vi "Rx Async.vi"(8 "error in (no error)":errorcluster, 10 "Dispatcher Interface in":refnum<class "Dispatcher Interface.lvclass">, 11 "Plugin in":refnum<class "Plugin.lvclass">) -> (0 "error out":errorcluster, 2 "Dispatcher Interface out":refnum<class "Dispatcher Interface.lvclass">, 3 "Plugin out":refnum<class "Plugin.lvclass">)   [LabVIEW 2017, in "DSF Core.lvlib" / "Plugin.lvclass"]
uses:
  Plugin.lvclass
  Interface/Dispatcher/Dispatcher Interface.lvclass
  Plugin.lvclass/Plugin.ctl
  Interface/Dispatcher/Command.ctl
  Transfer Group/Transfer Group.lvclass
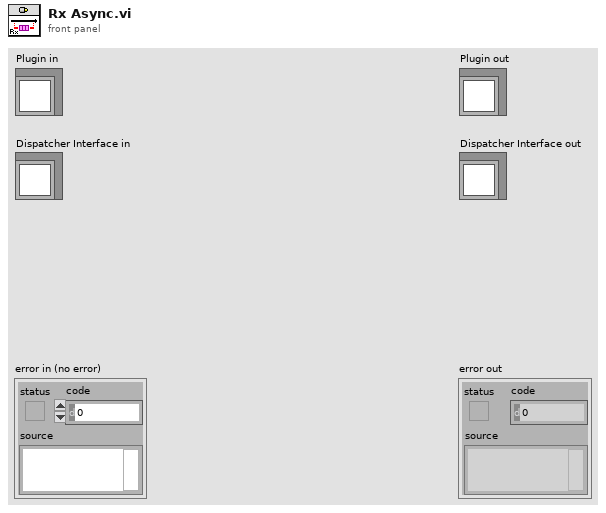
[diagram p1: front panel]
types:
  T1 = typedef "DSF Core.lvlib/Dispatcher Interface.lvclass/Command.ctl" = enum8{"Idle", "Start", "Rx", "Tx", "Set Inline Buffer", "Shutdown", "Error"}
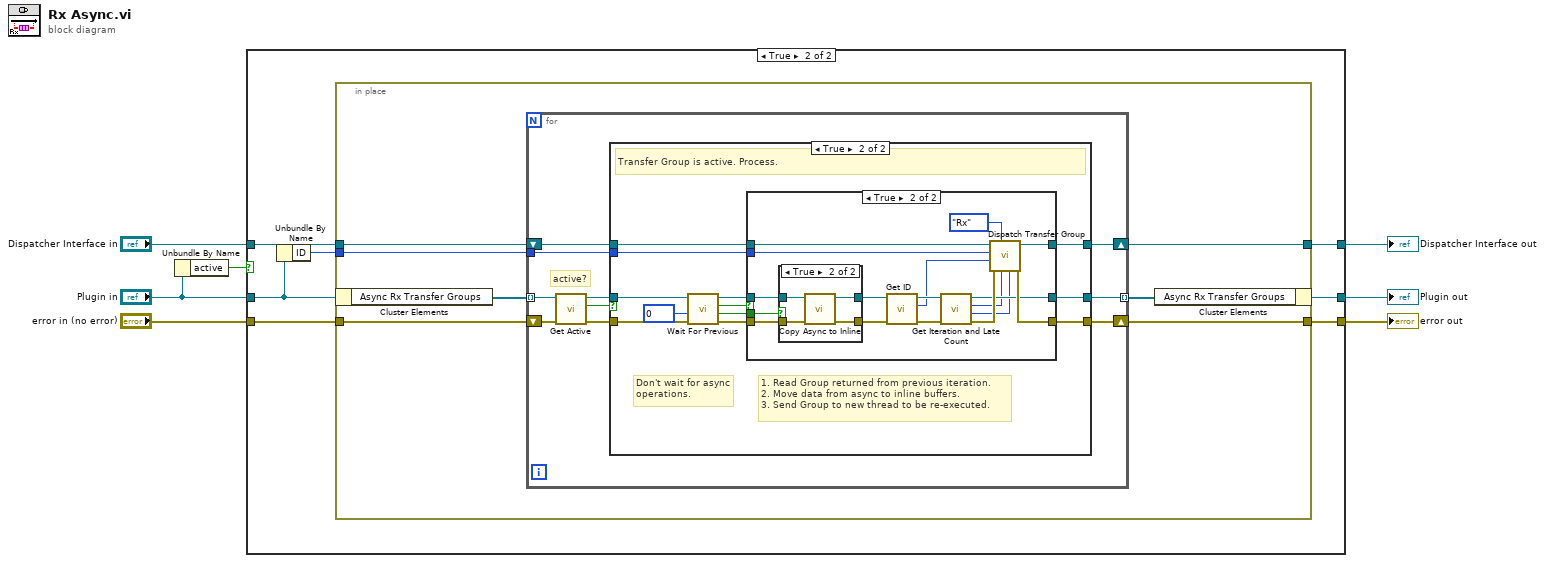
[diagram p0: block diagram]
diagram:
  n1 = Unbundle By Name("Plugin in") -> ("active"=w1:bool)
  n2 = case shown="True" w1 {
    tunnel: "error in (no error)" -> [w8 w17]
    tunnel: [w8 w16] -> w6
    tunnel: [w10 w15] -> w5
    tunnel: "Dispatcher Interface in" -> [w9 w14]
    tunnel: [w9 w13] -> w3
    tunnel: "Plugin in" -> [w10 w12]
    frame False {
    }
    frame True {
      n3 = Unbundle By Name(w12) -> ("ID"=w11:i32)
      n4 = in-place {
        in-place-border: w17 -> [w24]
        in-place-border: [w23] -> w16
        in-place-border: w14 -> [w20]
        in-place-border: [w19] -> w13
        in-place-border: w11 -> [w18]
        n5 = in-place-cluster #1(w12) -> ("Async Rx Transfer Groups"=w22:refnum<class "Transfer Group.lvclass">[])
        n6 = for {
          tunnel: w22 -> [w27] mode=indexing
          shift-right: [w33] -> w23
          shift-left: w24 -> [w32]
          tunnel: [w31] -> w21 mode=indexing
          shift-right: [w29] -> w19
          shift-left: w20 -> [w30]
          tunnel: w18 -> [w28]
          # "active?"
          n7 = call "Get Active.vi"("Transfer Group in"=w27) -> ("active"=w25:bool, "Transfer Group out"=w26:refnum<class "Transfer Group.lvclass">)  [unwired: 9 in]
          n8 = case shown="True" w25 {
            tunnel: [w36 w38] -> w33
            tunnel: w32 -> [w36 w47]
            tunnel: w26 -> [w35 w48]
            tunnel: [w35 w39] -> w31
            tunnel: w30 -> [w34 w42]
            tunnel: [w34 w43] -> w29
            tunnel: w28 -> [_ w41]
            frame False {
              # "Transfer Group is not active. Skip."
            }
            frame True {
              # "Don't wait for async operations."
              # "1. Read Group returned from previous iteration.\n2. Move data from async to inline buffers.\n3. Send Group to new thread to be re-executed."
              # "Transfer Group is active. Process."
              n9 = call "Wait For Previous.vi"("error in (no error)"=w47, "timeout in ms (0)"=0, "Transfer Group in"=w48) -> ("error out"=w44:errorcluster, "move data"=w37:bool, "ready"=w40:bool, "Transfer Group out"=w45:refnum<class "Transfer Group.lvclass">)  [unwired: 5 in]
              n10 = case shown="True" w40 {
                tunnel: w45 -> [w51 w67]
                tunnel: [w51 w59] -> w39
                tunnel: [w50 w60] -> w38
                tunnel: w44 -> [w50 w66]
                tunnel: [w49 w57] -> w43
                tunnel: w42 -> [w49 w56]
                tunnel: w41 -> [_ w55]
                tunnel: w37 -> [_ w54]
                frame False {
                }
                frame True {
                  n11 = case shown="True" w54 {
                    tunnel: w67 -> [w69 w73]
                    tunnel: w66 -> [w68 w72]
                    tunnel: [w69 w71] -> w52
                    tunnel: [w68 w70] -> w64
                    frame False {
                    }
                    frame True {
                      n12 = call "Copy Async to Inline.vi"("error in (no error)"=w72, "Transfer Group in"=w73) -> ("error out"=w70:errorcluster, "Transfer Group out"=w71:refnum<class "Transfer Group.lvclass">)  [unwired: 8 in]
                    }
                  }
                  n13 = call "Get ID.vi"("Transfer Group in"=w52) -> ("id"=w63:i32, "Transfer Group out"=w65:refnum<class "Transfer Group.lvclass">)  [unwired: 9 in]
                  n14 = call "Get Iteration and Late Count.vi"("error in (no error)"=w64, "Transfer Group in"=w65) -> ("error out"=w62:errorcluster, "late count"=w53:i32, "iteration"=w58:u64, "Transfer Group out"=w59:refnum<class "Transfer Group.lvclass">)  [unwired: 6 in]
                  n15 = call "Dispatch Transfer Group.vi"("Late Count"=w53, "Iteration"=w58, "command"=Command."Rx", "error in (no error)"=w62, "Transfer Group ID"=w63, "Plugin ID"=w55, "Dispatcher Interface in"=w56) -> ("error out"=w60:errorcluster, "Dispatcher Interface out"=w57:refnum<class "Dispatcher Interface.lvclass">)  [unwired: 3 in]
                }
              }
            }
          }
        }
        n16 = in-place-cluster #1("Async Rx Transfer Groups"=w21) -> (w15:refnum<class "Plugin.lvclass">)
      }
    }
  }
  "error out" <- w6
  "Plugin out" <- w5
  "Dispatcher Interface out" <- w3
